vi "Spartan Client.vi"() -> ()   [LabVIEW 2011]
uses:
  <vilib>/Utility/miscctls.llb/LVPointTypeDef.ctl
  OpenG.LIB/file/file.llb/Convert File Extension (Path)__ogtk.vi
  client.lib/Spartan Client Version.vi
  <vilib>/Platform/browser.llb/Open URL in Default Browser (string).vi
  Program Files/National Instruments/LabVIEW 2011/resource/lvsound.dll
  Program Files/National Instruments/LabVIEW 2011/resource/lvanlys.dll
panel:
  out "Server":string
  out "Port":u16
  in  "Tab":enum32{"Local", "Comm"}(tab)
  out "Local":string
  out "Comm":string
  out "blinky":bool
  in  "weblink":bool
  in  "Boolean":bool
  out "Client":string
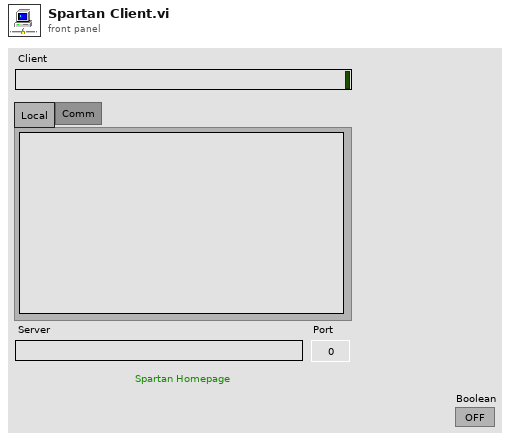
[diagram p1: front panel]
types:
  T1 = enum32{"SW_SHOWDEFAULT", "SW_FORCEMINIMIZE", "SW_HIDE", "SW_MAXIMIZE", "SW_RESTORE", "SW_SHOW", "SW_SHOWMAXIMIZED", "SW_SHOWMINIMIZED", "SW_SHOWMINNOACTIVE", "SW_SHOWNA", "SW_SHOWNOACTIVATE", "SW_SHOWNORMAL"}
  T2 = typedef "LVPointTypeDef.ctl" = cluster{"Horizontal":i16, "Vertical":i16}
  T3 = typedef "OGAB Version.ctl" = cluster{"Version":string, "Build Number":u32, "Build Date/Time":dbl}
  T4 = typedef "hWnd.ctl" = refnum<k1>
  T5 = typedef "siwutil32.ctl" = refnum<k7>
  T6 = typedef "sizeaction.ctl" = enum32{"Minimized", "Maximized", "Resized"}
  T7 = enum32{"invalid app kind", "Development System", "Run Time System", "Student Edition", "Embedded LabVIEW", "Evaluation", "Custom"}
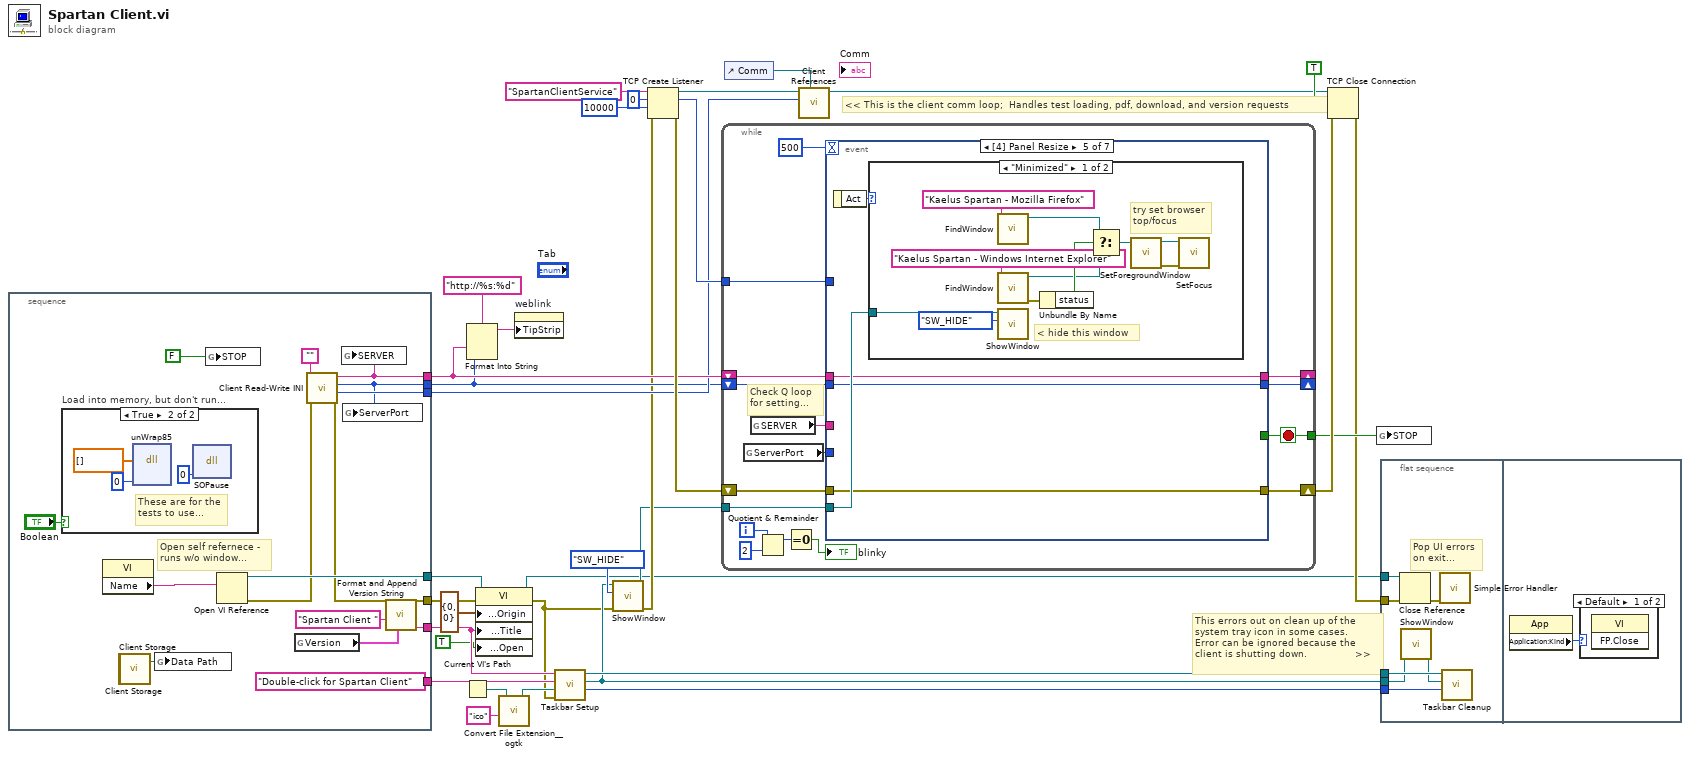
[diagram p0: block diagram]
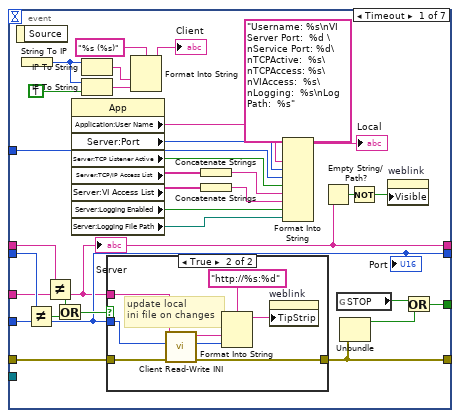
[diagram p3: hidden frame]
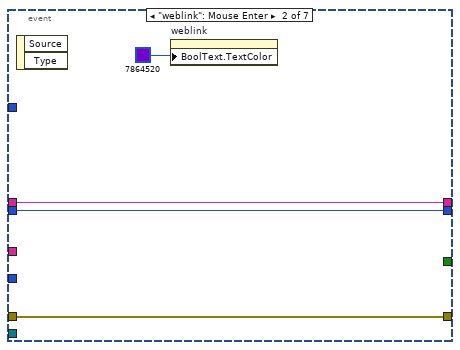
[diagram p5: hidden frame]
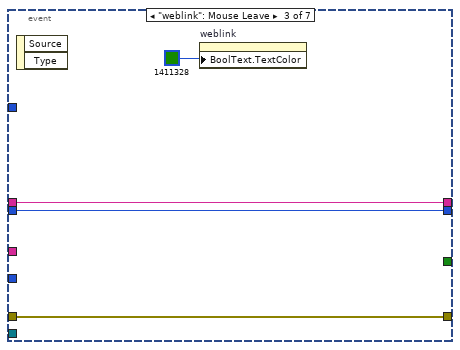
[diagram p6: hidden frame]
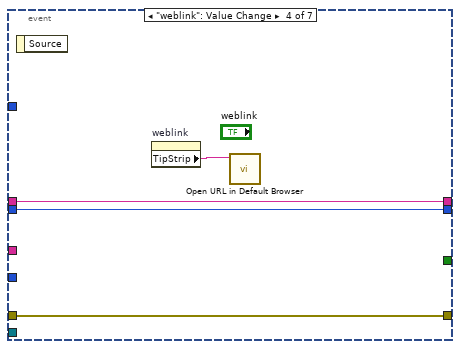
[diagram p7: hidden frame]
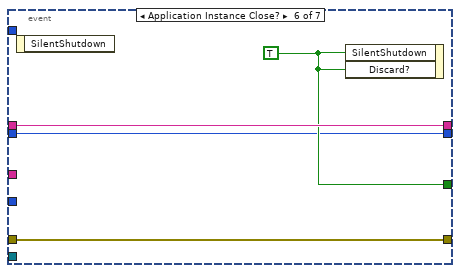
[diagram p9: hidden frame]
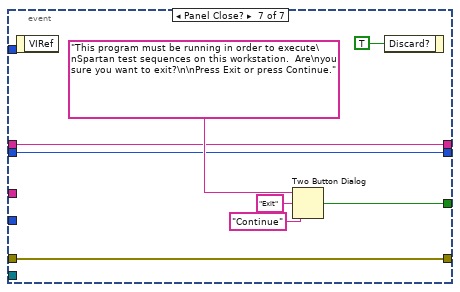
[diagram p10: hidden frame]
diagram:
  # "<< This is the client comm loop;  Handles test loading, pdf, download, and version requests"
  # "This errors out on clean up of the\nsystem tray icon in some cases.\nError can be ignored because the\nclient is shutting down.                >>"
  n1 = stacked-sequence {
    tunnel: [w44] -> w34
    tunnel: ["Double-click for Spartan Client" ("format string")] -> w33
    tunnel: [w43] -> w29
    tunnel: [w47] -> w27
    tunnel: [w45] -> w9
    tunnel: [w40] -> w8
    tunnel: [w37] -> w7
    frame #0 {
      # "Open self refernece -\nruns w/o window..."
      n2 = case "Load into memory, but don't run..." shown="True" "Boolean" {
        frame False {
        }
        frame True {
          # "These are for the\ntests to use..."
          n3 = dll-call lib="C:/Program Files/National Instruments/LabVIEW 2011/resource/lvanlys.*" fn="unWrap85" label="lvanlys.dll"("Phase"=dbl[] [], "phase unit"=0) -> ()  [unwired: 4 in, 4 out]
          n4 = dll-call lib="C:/Program Files/National Instruments/LabVIEW 2011/resource/lvsound.*" fn="SOPause" label="lvsound.dll"("taskID"=u32 0) -> ()  [unwired: 4 in, 3 out]
        }
      }
      n5 = property class="VI"() -> ("Name"=w42:string)  [unwired: 2 in, 2 out]
      n6 = call "Client Storage.vi"() -> ()  [unwired: 3 in, 1 out]
      n7 = call "Client Storage.vi"() -> ("Client Storage Path"=w35:path)  [unwired: 3 in]
      n8 = global write "Spartan Client Version.vi" "Data Path"(w35) -> ()
      n9 = global write "Spartan Client Version.vi" "STOP"(FALSE) -> ()
      n10 = Open VI Reference(vi path=w42) -> (vi reference=w47:refnum<vi>, error out=w41:errorcluster)  [unwired: 1 in, 4 out]
      n11 = global read "Spartan Client Version.vi" "Version"() -> (w36:T3)
      n12 = call "Client Read-Write INI.vi"("error in (no error)"=w41, "ServerName (Empty - Read)"="") -> ("error out"=w43:errorcluster, "Test Timeout (ms)"=w40:i32, "ServerPort out"=w37:u16, "ServerName Out"=w45:string)  [unwired: 1 in, 5 out]
      n13 = global write "Spartan Client Version.vi" "SERVER"(w45) -> ()
      n14 = global write "Spartan Client Version.vi" "ServerPort"(w37) -> ()
      n15 = call "Format and Append Version String.vi"("Version"=w36, "String (Empty)"="Spartan Client " ("format string")) -> ("String with Version & Build"=w44:string)  [unwired: 1 in, 8 out]
    }
  }
  n16 = Current VI's Path() -> (path=w14:path)
  n17 = Format Into String(format string="http://%s:%d", w9, w7) -> (resulting string=w11:string)  [unwired: 2 in, 1 out]
  n18 = property class="VI"(reference=w27, error in=w29, "Front Panel Window:Origin"=T2 {"Horizontal"=0, "Vertical"=0}, "Front Panel Window:Title"=w34, "Front Panel Window:Open"=TRUE) -> (reference out=w1:refnum<vi>, error out=w2:errorcluster)
  n19 = call-poly "Convert File Extension__ogtk.vi"("new ending (none)"="ico", "file name"=w14) -> ("new filename"=w15:path)  [unwired: 1 out]
  n20 = property on="weblink" class="Bool"("TipStrip"=w11) -> ()  [unwired: 2 in, 2 out]
  n21 = call "Taskbar Setup.vi"("error in (no error)"=w2, "DEV Icon Path (empty)"=w15, "Tooltip Text (\"\")"=w33, "Window Name (\"\")"=w34) -> ("hIcon"=w30:i32, "hWnd"=w4:T4, "siwutil32"=w31:T5)  [unwired: 1 out]
  n22 = call "ShowWindow.vi"("error in (no error)"=w2, "nCmdShow\n(SW_SHOWNORMAL)"=T1."SW_HIDE" ("nCmdShow\n(SW_SHOWNORMAL)"), "hWnd (NULL)"=w4) -> ("error out"=w5:errorcluster, "dup hWnd"=w3:T4)  [unwired: 7 out]
  n23 = TCP Create Listener(8:w5, 9:10000 ("timeout ms (25000)"), 10:u16 0 ("port"), 11:"SpartanClientService" ("service name")) -> (0:w23:errorcluster, 2:w21:u16, 3:w22:refnum<k5>)  [unwired: 1 out]
  n24 = while {
    tunnel: w3 -> [w67]
    shift-right: [w64] -> _
    shift-left: w9 -> [w65]
    shift-right: [w63] -> w18
    shift-left: w23 -> [w59]
    tunnel: w21 -> [w60]
    tunnel: [w56] -> w17
    shift-right: [w53] -> _
    shift-left: w7 -> [w54]
    i -> [w62]
    stop <- w56 stop-if-true
    # "Check Q loop\nfor setting..."
    n25 = global read "Spartan Client Version.vi" "ServerPort"() -> (w55:u16)
    n26 = global read "Spartan Client Version.vi" "SERVER"() -> (w66:string)
    n27 = Quotient & Remainder(x=w62, y=2) -> (x-y*floor(x/y)=w57:i32)  [unwired: 1 out]
    n28 = Equal To 0?(x=w57) -> (x = 0?=→"blinky":bool)
    n29 = event shown="[4] Panel Resize" {
      selector: _ -> [_ _ _ _ _ _ _]
      dyn-events: _ -> [_ _ _ _ _ _ _]
      timeout: 500 -> [_ _ _ _ _ _ _]
      tunnel: w59 -> [w84 w113 w117 w121 w123 w140 w146]
      tunnel: [w81 w113 w117 w121 w123 w140 w146] -> w63
      tunnel: w67 -> [_ _ _ _ w125 _ _]
      tunnel: w66 -> [w69 _ _ _ _ _ _]
      tunnel: w65 -> [w85 w112 w116 w120 w124 w141 w147]
      tunnel: [w69 w112 w116 w120 w124 w141 w147] -> w64
      tunnel: w60 -> [w80 _ _ _ _ _ _]
      tunnel: [w77 _ _ _ _ w139 w145] -> w56
      tunnel: w55 -> [w70 _ _ _ _ _ _]
      tunnel: w54 -> [w71 w110 w114 w118 w122 w138 w142]
      tunnel: [w70 w110 w114 w118 w122 w138 w142] -> w53
      event Timeout {
        n30 = event-data() -> ()  [unwired: 2 out]
        n31 = String To IP() -> (0:w99:u32)  [unwired: 1 out]
        n32 = Not Equal?(x=w71, y=w70) -> (x != y?=w75:bool)
        n33 = Not Equal?(x=w85, y=w69) -> (x != y?=w74:bool)
        n34 = Or(x=w74, y=w75) -> (x .or. y?=w73:bool)
        n35 = property class="App"() -> ("Application:User Name"=w76:string, "Server:Port"=w93:u32, "Server:TCP Listener Active"=w92:bool, "Server:TCP/IP Access List"=w91:string[], "Server:VI Access List"=w88:string[], "Server:Logging Enabled"=w86:bool, "Server:Logging File Path"=w72:path)  [unwired: 2 in, 2 out]
        n36 = IP To String(2:w99) -> (0:w97:string)  [unwired: 1 out]
        n37 = IP To String(1:TRUE, 2:w99) -> (0:w96:string)
        n38 = case shown="True" w73 {
          tunnel: w69 -> [_ w109]
          tunnel: w84 -> [w101 w108]
          tunnel: [w101 w107] -> w81
          tunnel: w70 -> [_ w103]
          frame False {
          }
          frame True {
            # "update local\nini file on changes"
            n39 = call "Client Read-Write INI.vi"("error in (no error)"=w108, "ServerPort (80)"=w103, "ServerName (Empty - Read)"=w109) -> ("error out"=w107:errorcluster, "ServerPort out"=w102:u16, "ServerName Out"=w106:string)  [unwired: 6 out]
            n40 = Format Into String(format string="http://%s:%d", w106, w102) -> (resulting string=w104:string)  [unwired: 2 in, 1 out]
            n41 = property on="weblink" class="Bool"("TipStrip"=w104) -> ()  [unwired: 2 in, 2 out]
          }
        }
        n42 = Format Into String(format string="%s (%s)", w97, w96) -> (resulting string=→"Client":string)  [unwired: 2 in, 1 out]
        n43 = Concatenate Strings(w91) -> (w90:string)
        n44 = Concatenate Strings(w88) -> (w89:string)
        n45 = Format Into String(format string="Username: %s\nVI Server Port:  %d \nService Port: %d\nTCPActive:  %s\nTCPAccess: %s\nVIAccess:  %s\nLogging:  %s\nLog Path:  %s", w76, w93, w80, w92, w90, w89, w86, w72) -> (resulting string=→"Local":string)  [unwired: 2 in, 1 out]
        n46 = Empty String/Path?(string/path=w69) -> (empty?=w83:bool)
        n47 = global read "Spartan Client Version.vi" "STOP"() -> (w79:bool)
        n48 = Unbundle(w81) -> ("status"=w78:bool)  [unwired: 2 out]
        n49 = Not(x=w83) -> (.not. x?=w82:bool)
        n50 = property on="weblink" class="Bool"("Visible"=w82) -> ()  [unwired: 2 in, 2 out]
        n51 = Or(x=w79, y=w78) -> (x .or. y?=w77:bool)
        "Port" <- w70
        "Server" <- w69
      }
      event "weblink": Mouse Enter {
        n52 = event-data() -> ()  [unwired: 3 out]
        n53 = property on="weblink" class="Bool"("BoolText.TextColor"=u32 7864520) -> ()  [unwired: 2 in, 2 out]
      }
      event "weblink": Mouse Leave {
        n54 = event-data() -> ()  [unwired: 3 out]
        n55 = property on="weblink" class="Bool"("BoolText.TextColor"=u32 1411328) -> ()  [unwired: 2 in, 2 out]
      }
      event "weblink": Value Change {
        n56 = event-data() -> ()  [unwired: 2 out]
        n57 = property on="weblink" class="Bool"() -> ("TipStrip"=w119:string)  [unwired: 2 in, 2 out]
        n58 = call-poly <vilib>:"Open URL in Default Browser.vi"("URL"=w119) -> ()  [unwired: 1 in, 6 out]
      }
      event Panel Resize {
        n59 = event-data() -> ("Act"=w126:T6)  [unwired: 1 out]
        n60 = case shown="\"Minimized\"" w126 {
          tunnel: w125 -> [w137 _]
          frame "Minimized" {
            # "< hide this window"
            # "try set browser\ntop/focus"
            n61 = call "FindWindow.vi"("window name (\"\")"="Kaelus Spartan - Mozilla Firefox" ("window name (\"\")")) -> ("hWnd"=w134:T4)  [unwired: 1 in, 7 out]
            n62 = call "FindWindow.vi"("window name (\"\")"="Kaelus Spartan - Windows Internet Explorer" ("window name (\"\")")) -> ("error out"=w132:errorcluster, "hWnd"=w131:T4)  [unwired: 1 in, 6 out]
            n63 = call "ShowWindow.vi"("nCmdShow\n(SW_SHOWNORMAL)"=T1."SW_HIDE" ("nCmdShow\n(SW_SHOWNORMAL)"), "hWnd (NULL)"=w137) -> ()  [unwired: 1 in, 9 out]
            n64 = Unbundle By Name(w132) -> ("status"=w133:bool)
            n65 = Select(t=w134, s=w133, f=w131) -> (s? t:f=w127:T4)
            n66 = call "SetForegroundWindow.vi"("hWnd (NULL)"=w127) -> ("error out"=w128:errorcluster, "dup hWnd"=w129:T4)  [unwired: 1 in, 8 out]
            n67 = call "SetFocus.vi"("error in (no error)"=w128, "hWnd (NULL)"=w129) -> ()  [unwired: 10 out]
          }
          frame Default {
          }
        }
      }
      event Application Instance Close? {
        w139 = TRUE
        n68 = event-data() -> ()  [unwired: 2 out]
        n69 = event-data("SilentShutdown"=w139, "Discard?"=w139) -> ()  [unwired: 1 in, 1 out]
      }
      event Panel Close? {
        n70 = event-data() -> ()  [unwired: 2 out]
        n71 = Two Button Dialog(message="This program must be running in order to execute\nSpartan test sequences on this workstation.  Are\nyou sure you want to exit?\n\nPress Exit or press Continue.", 1:"Continue" ("T button name (\"OK\")"), 2:"Exit" ("T button name (\"OK\")")) -> (T button?=w145:bool)
        n72 = event-data("Discard?"=TRUE) -> ()  [unwired: 1 in, 1 out]
      }
    }
  }
  n73 = control-ref of="Comm"() -> (w13:refnum<vi>)
  n74 = call "Client References.vi"("Comm ref"=w13, "TestTimeout (0 ms)"=w8, "tcp listener ref"=w22) -> ("dup tcp listener ref"=w19:refnum<k5>)  [unwired: 1 in, 7 out]
  n75 = TCP Close Connection(connection ID=w19, abort (F)=TRUE, error in (no error)=w18) -> (error out=w12:errorcluster)  [unwired: 1 out]
  n76 = global write "Spartan Client Version.vi" "STOP"(w17) -> ()
  n77 = flat-sequence {
    tunnel: w12 -> [w153]
    tunnel: w31 -> [w156]
    tunnel: w4 -> [w155]
    tunnel: w30 -> [w154]
    tunnel: w1 -> [w152]
    frame #0 {
      # "Pop UI errors\non exit..."
      n78 = Close Reference(reference=w152, error in (no error)=w153) -> (error out=w150:errorcluster)
      n79 = call "ShowWindow.vi"("hWnd (NULL)"=w155) -> ("dup hWnd"=w151:T4)  [unwired: 2 in, 8 out]
      n80 = call <vilib>:"Simple Error Handler.vi"("error in (no error)"=w150) -> ()  [unwired: 1 in, 8 out]
      n81 = call "Taskbar Cleanup.vi"("hIcon"=w154, "hWnd"=w151, "siwutil32"=w156) -> ()  [unwired: 1 in, 4 out]
    }
    frame #1 {
      n82 = property class="App"() -> ("Application:Kind"=w157:T7)  [unwired: 2 in, 2 out]
      n83 = case shown="Default" w157 {
        frame Default {
          n84 = invoke class="VI" method="FP.Close"() -> ()  [unwired: 3 in, 3 out]
        }
        frame "Development System" {
        }
      }
    }
  }
